vi "Destroy.vi"(8 "error in (no error)":errorcluster, 11 "Boolean In":refnum<class "Boolean.lvclass">) -> (0 "error out":errorcluster, 3 "Boolean Out":refnum<class "Boolean.lvclass">)   [LabVIEW 2015, in "Front Panel Publisher.lvlib" / "Boolean.lvclass"]
uses:
  Boolean.lvclass
  Control_class/Control.lvclass
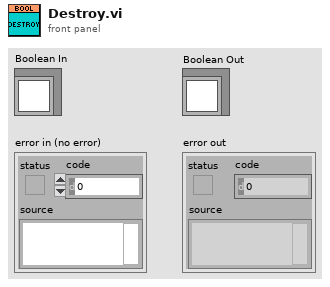
[diagram p1: front panel]
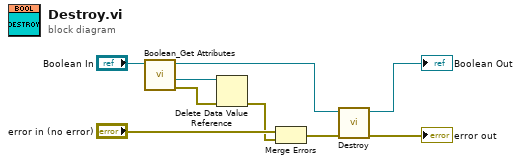
[diagram p0: block diagram]
diagram:
  n1 = call "Boolean_Get Attributes.vi"("Boolean In"="Boolean In") -> ("error out"=w8:errorcluster, "DataRef"=w7:refnum<data-value>, "Boolean Out"=w3:refnum<class "Boolean.lvclass">)  [unwired: 7 in, 1 out]
  n2 = Delete Data Value Reference(data value reference=w7, error in=w8) -> (error out=w5:errorcluster)  [unwired: 1 out]
  n3 = Merge Errors("error in (no error)", w5) -> (w4:errorcluster)
  n4 = call-parent "Destroy.vi"("error in (no error)"=w4, "Control In"=w3) -> ("error out"=→"error out":errorcluster, "Control Out"=→"Boolean Out":refnum<class "Boolean.lvclass">)  [unwired: 8 in]
